vi "EOL Main.vi"() -> ()   [LabVIEW 2018]
uses:
  02.Type Def's/station motion data indicator.ctl
  02.Type Def's/Screen Motion Data.ctl
  02.Type Def's/Pass Fail Control.ctl
  02.Type Def's/station hmi.ctl
  02.Type Def's/lvdt name val pair.ctl
  02.Type Def's/individual station status.ctl
  02.Type Def's/repair station status.ctl
panel:
  in  "NVH Status":bool
  in  "Sunshade Graphs":bool
  out "ms":dbl
  out "All Stations Stopped":bool
  in  "st3":bool
  in  "st0":bool
  in  "O'Scope Data":bool
  in  "Pretty Graphs":bool
  in  "Barcode":bool
  in  "st2":bool
  in  "st1":bool
  in  "All Stations":bool
  in  "Configuration":bool
  in  "Exit Program":bool
  out "Time":string
  out "Date":string
  in  "Main Tab Control":T1(tab)
  in  "Red-Rabbit Mode 3":bool
  in  "Route to Repair st 3":bool
  in  "Abort Test st 3":bool
  in  "Start Test st 3":bool
  in  "Manual Control st 3":bool
  out "all station status st 0":T2={"Error Table Br"=[], "Pass / Fail"=9868950, "Cycle Time Br"=0.0, "Sunroof Barcode"="", "Pallet Number"="", "Part Type"="", "Current Step Br"="", "Application Status"="", "Station Name"="", "Database LVDT's Data Out"=[], "NVH System"=FALSE, "Date"="", "Time"=""} {"Database LVDT's Data Out"."value" format="%.2f"; "Cycle Time Br" format="%#.2g"}
  out "all station status st 3":T2={"Error Table Br"=[], "Pass / Fail"=9868950, "Cycle Time Br"=0.0, "Sunroof Barcode"="", "Pallet Number"="", "Part Type"="", "Current Step Br"="", "Application Status"="", "Station Name"="", "Database LVDT's Data Out"=[], "NVH System"=FALSE, "Date"="", "Time"=""} {"Database LVDT's Data Out"."value" format="%.2f"; "Cycle Time Br" format="%#.2g"}
  in  "Red-Rabbit Mode 2":bool
  in  "Route to Repair st 2":bool
  in  "Abort Test st 2":bool
  in  "Start Test st 2":bool
  in  "Manual Control st 2":bool
  out "all station status st 2":T2={"Error Table Br"=[], "Pass / Fail"=9868950, "Cycle Time Br"=0.0, "Sunroof Barcode"="", "Pallet Number"="", "Part Type"="", "Current Step Br"="", "Application Status"="", "Station Name"="", "Database LVDT's Data Out"=[], "NVH System"=FALSE, "Date"="", "Time"=""} {"Database LVDT's Data Out"."value" format="%.2f"; "Cycle Time Br" format="%#.2g"}
  in  "Red-Rabbit Mode 1":bool
  in  "Route to Repair st 1":bool
  in  "Abort Test st 1":bool
  in  "Start Test st 1":bool
  in  "Manual Control st 1":bool
  in  "Red-Rabbit Mode 0":bool
  out "Repair Station:":T4
  out "Main Title":string=" - All Stations Status"
  in  "Route to Repair st 0":bool
  in  "Abort Test st 0":bool
  in  "Start Test st 0":bool
  in  "Manual Control st 0":bool
  in  "Start Test Re":bool
  in  "Manual Control Repair":bool
  out "all station status st 1":T2={"Error Table Br"=[], "Pass / Fail"=9868950, "Cycle Time Br"=0.0, "Sunroof Barcode"="", "Pallet Number"="", "Part Type"="", "Current Step Br"="", "Application Status"="", "Station Name"="", "Database LVDT's Data Out"=[], "NVH System"=FALSE, "Date"="", "Time"=""} {"Database LVDT's Data Out"."value" format="%.2f"; "Cycle Time Br" format="%#.2g"}
  in  "Tab Control 0":enum32{"Motion Current Data", "Motion Data"}(tab)
  out "Waveform Graph st 0":dbl[](graph)
  out "Motion Data st 0":T5={"Shade Close Limits"={"Noise Test"=enum."Not Tested", "Avg Current"=0.0, "Run Time"=0.0, "Speed"=0.0, "Position"=enum."Not Tested"}, "Shade Close Data 2"={"Noise Test"=enum."Not Tested", "Avg Current"=0.0, "Run Time"=0.0, "Speed"=0.0, "Position"=enum."Not Tested"}, "Shade Open Limits"={"Noise Test"=enum."Not Tested", "Avg Current"=5.0, "Run Time"=5.0, "Speed"=0.0, "Position"=enum."Not Tested"}, "Shade Open Data"={"Noise Test"=enum."Not Tested", "Avg Current"=0.0, "Run Time"=0.0, "Speed"=0.0, "Position"=enum."Not Tested"}, "Vent Close Limits"={"Noise Test"=enum."Not Tested", "Avg Current"=0.0, "Run Time"=0.0, "Speed"=0.0, "Position"=enum."Not Tested"}, "Vent Close Data"={"Noise Test"=enum."Not Tested", "Avg Current"=0.0, "Run Time"=0.0, "Speed"=0.0, "Position"=enum."Not Tested"}, "Vent Open Limits"={"Noise Test"=enum."Not Tested", "Avg Current"=0.0, "Run Time"=0.0, "Speed"=0.0, "Position"=enum."Not Tested"}, "Vent Open Data"={"Noise Test"=enum."Not Tested", "Avg Current"=0.0, "Run Time"=0.0, "Speed"=0.0, "Position"=enum."Not Tested"}, "Slide Close Limits"={"Noise Test"=enum."Not Tested", "Avg Current"=0.0, "Run Time"=0.0, "Speed"=0.0, "Position"=enum."Not Tested"}, "Slide Close Data"={"Noise Test"=enum."Not Tested", "Avg Current"=0.0, "Run Time"=0.0, "Speed"=0.0, "Position"=enum."Not Tested"}, "Slide Open Limits"={"Noise Test"=enum."Not Tested", "Avg Current"=0.0, "Run Time"=0.0, "Speed"=0.0, "Position"=enum."Not Tested"}, "Slide Open Data"={"Noise Test"=enum."Not Tested", "Avg Current"=0.0, "Run Time"=0.0, "Speed"=0.0, "Position"=enum."Not Tested"}} {"Shade Close Limits"."Speed" format="%.2g"; "Shade Close Limits"."Run Time" format="%.2g"; "Shade Close Limits"."Avg Current" format="%.2g"; "Shade Close Data 2"."Speed" format="%.2g"; "Shade Close Data 2"."Run Time" format="%.2g"; "Shade Close Data 2"."Avg Current" format="%.2g"; "Shade Open Limits"."Speed" format="%.2g"; "Shade Open Limits"."Run Time" format="%.2g"; "Shade Open Limits"."Avg Current" format="%.2g"; "Shade Open Data"."Speed" format="%.2g"; "Shade Open Data"."Run Time" format="%.2g"; "Shade Open Data"."Avg Current" format="%.2g"; "Vent Close Limits"."Speed" format="%.2g"; "Vent Close Limits"."Run Time" format="%.2g"; "Vent Close Limits"."Avg Current" format="%.2g"; "Vent Close Data"."Speed" format="%.2g"; "Vent Close Data"."Run Time" format="%.2g"; "Vent Close Data"."Avg Current" format="%.2g"; "Vent Open Limits"."Speed" format="%.2g"; "Vent Open Limits"."Run Time" format="%.2g"; "Vent Open Limits"."Avg Current" format="%.2g"; "Vent Open Data"."Speed" format="%.2g"; "Vent Open Data"."Run Time" format="%.2g"; "Vent Open Data"."Avg Current" format="%.2g"; "Slide Close Limits"."Speed" format="%.2g"; "Slide Close Limits"."Run Time" format="%.2g"; "Slide Close Limits"."Avg Current" format="%.2g"; "Slide Close Data"."Speed" format="%.2g"; "Slide Close Data"."Run Time" format="%.2g"; "Slide Close Data"."Avg Current" format="%.2g"; "Slide Open Limits"."Speed" format="%.2g"; "Slide Open Limits"."Run Time" format="%.2g"; "Slide Open Limits"."Avg Current" format="%.2g"; "Slide Open Data"."Speed" format="%.2g"; "Slide Open Data"."Run Time" format="%.2g"; "Slide Open Data"."Avg Current" format="%.2g"}
  out "Individual Station Status st 0":T8
  in  "Tab Control 1":enum32{"Motion Current Data", "Motion Data"}(tab)
  out "Waveform Graph st 1":dbl[](graph)
  out "Motion Data st 1":T5 {"Shade Close Limits"."Speed" format="%.2g"; "Shade Close Limits"."Run Time" format="%.2g"; "Shade Close Limits"."Avg Current" format="%.2g"; "Shade Close Data 2"."Speed" format="%.2g"; "Shade Close Data 2"."Run Time" format="%.2g"; "Shade Close Data 2"."Avg Current" format="%.2g"; "Shade Open Limits"."Speed" format="%.2g"; "Shade Open Limits"."Run Time" format="%.2g"; "Shade Open Limits"."Avg Current" format="%.2g"; "Shade Open Data"."Speed" format="%.2g"; "Shade Open Data"."Run Time" format="%.2g"; "Shade Open Data"."Avg Current" format="%.2g"; "Vent Close Limits"."Speed" format="%.2g"; "Vent Close Limits"."Run Time" format="%.2g"; "Vent Close Limits"."Avg Current" format="%.2g"; "Vent Close Data"."Speed" format="%.2g"; "Vent Close Data"."Run Time" format="%.2g"; "Vent Close Data"."Avg Current" format="%.2g"; "Vent Open Limits"."Speed" format="%.2g"; "Vent Open Limits"."Run Time" format="%.2g"; "Vent Open Limits"."Avg Current" format="%.2g"; "Vent Open Data"."Speed" format="%.2g"; "Vent Open Data"."Run Time" format="%.2g"; "Vent Open Data"."Avg Current" format="%.2g"; "Slide Close Limits"."Speed" format="%.2g"; "Slide Close Limits"."Run Time" format="%.2g"; "Slide Close Limits"."Avg Current" format="%.2g"; "Slide Close Data"."Speed" format="%.2g"; "Slide Close Data"."Run Time" format="%.2g"; "Slide Close Data"."Avg Current" format="%.2g"; "Slide Open Limits"."Speed" format="%.2g"; "Slide Open Limits"."Run Time" format="%.2g"; "Slide Open Limits"."Avg Current" format="%.2g"; "Slide Open Data"."Speed" format="%.2g"; "Slide Open Data"."Run Time" format="%.2g"; "Slide Open Data"."Avg Current" format="%.2g"}
  out "Individual Station Status st 1":T8
  in  "Tab Control 2":enum32{"Motion Current Data", "Motion Data"}(tab)
  out "Waveform Graph st 2":dbl[](graph)
  out "Motion Data st 2":T5={"Shade Close Limits"={"Noise Test"=enum."Not Tested", "Avg Current"=0.0, "Run Time"=0.0, "Speed"=0.0, "Position"=enum."Not Tested"}, "Shade Close Data 2"={"Noise Test"=enum."Not Tested", "Avg Current"=0.0, "Run Time"=0.0, "Speed"=0.0, "Position"=enum."Not Tested"}, "Shade Open Limits"={"Noise Test"=enum."Not Tested", "Avg Current"=5.0, "Run Time"=5.0, "Speed"=0.0, "Position"=enum."Not Tested"}, "Shade Open Data"={"Noise Test"=enum."Not Tested", "Avg Current"=0.0, "Run Time"=0.0, "Speed"=0.0, "Position"=enum."Not Tested"}, "Vent Close Limits"={"Noise Test"=enum."Not Tested", "Avg Current"=0.0, "Run Time"=0.0, "Speed"=0.0, "Position"=enum."Not Tested"}, "Vent Close Data"={"Noise Test"=enum."Not Tested", "Avg Current"=0.0, "Run Time"=0.0, "Speed"=0.0, "Position"=enum."Not Tested"}, "Vent Open Limits"={"Noise Test"=enum."Not Tested", "Avg Current"=0.0, "Run Time"=0.0, "Speed"=0.0, "Position"=enum."Not Tested"}, "Vent Open Data"={"Noise Test"=enum."Not Tested", "Avg Current"=0.0, "Run Time"=0.0, "Speed"=0.0, "Position"=enum."Not Tested"}, "Slide Close Limits"={"Noise Test"=enum."Not Tested", "Avg Current"=0.0, "Run Time"=0.0, "Speed"=0.0, "Position"=enum."Not Tested"}, "Slide Close Data"={"Noise Test"=enum."Not Tested", "Avg Current"=0.0, "Run Time"=0.0, "Speed"=0.0, "Position"=enum."Not Tested"}, "Slide Open Limits"={"Noise Test"=enum."Not Tested", "Avg Current"=0.0, "Run Time"=0.0, "Speed"=0.0, "Position"=enum."Not Tested"}, "Slide Open Data"={"Noise Test"=enum."Not Tested", "Avg Current"=0.0, "Run Time"=0.0, "Speed"=0.0, "Position"=enum."Not Tested"}} {"Shade Close Limits"."Speed" format="%.2g"; "Shade Close Limits"."Run Time" format="%.2g"; "Shade Close Limits"."Avg Current" format="%.2g"; "Shade Close Data 2"."Speed" format="%.2g"; "Shade Close Data 2"."Run Time" format="%.2g"; "Shade Close Data 2"."Avg Current" format="%.2g"; "Shade Open Limits"."Speed" format="%.2g"; "Shade Open Limits"."Run Time" format="%.2g"; "Shade Open Limits"."Avg Current" format="%.2g"; "Shade Open Data"."Speed" format="%.2g"; "Shade Open Data"."Run Time" format="%.2g"; "Shade Open Data"."Avg Current" format="%.2g"; "Vent Close Limits"."Speed" format="%.2g"; "Vent Close Limits"."Run Time" format="%.2g"; "Vent Close Limits"."Avg Current" format="%.2g"; "Vent Close Data"."Speed" format="%.2g"; "Vent Close Data"."Run Time" format="%.2g"; "Vent Close Data"."Avg Current" format="%.2g"; "Vent Open Limits"."Speed" format="%.2g"; "Vent Open Limits"."Run Time" format="%.2g"; "Vent Open Limits"."Avg Current" format="%.2g"; "Vent Open Data"."Speed" format="%.2g"; "Vent Open Data"."Run Time" format="%.2g"; "Vent Open Data"."Avg Current" format="%.2g"; "Slide Close Limits"."Speed" format="%.2g"; "Slide Close Limits"."Run Time" format="%.2g"; "Slide Close Limits"."Avg Current" format="%.2g"; "Slide Close Data"."Speed" format="%.2g"; "Slide Close Data"."Run Time" format="%.2g"; "Slide Close Data"."Avg Current" format="%.2g"; "Slide Open Limits"."Speed" format="%.2g"; "Slide Open Limits"."Run Time" format="%.2g"; "Slide Open Limits"."Avg Current" format="%.2g"; "Slide Open Data"."Speed" format="%.2g"; "Slide Open Data"."Run Time" format="%.2g"; "Slide Open Data"."Avg Current" format="%.2g"}
  out "Individual Station Status st 2":T8
  out "Sunshade Servo Data Open":dbl[](graph)
  out "AP Data Graph":i16[][](graph)
  in  "AP Data":path
  in  "Update AP Data":bool
  out "Sunshade Servo Data Close":dbl[](graph)
  out "Individual Station Status st 3":T8
  in  "Tab Control 3":enum32{"Motion Current Data", "Motion Data"}(tab)
  out "Waveform Graph st 3":dbl[](graph)
  out "Motion Data st 3":T5 {"Shade Close Limits"."Speed" format="%.2g"; "Shade Close Limits"."Run Time" format="%.2g"; "Shade Close Limits"."Avg Current" format="%.2g"; "Shade Close Data 2"."Speed" format="%.2g"; "Shade Close Data 2"."Run Time" format="%.2g"; "Shade Close Data 2"."Avg Current" format="%.2g"; "Shade Open Limits"."Speed" format="%.2g"; "Shade Open Limits"."Run Time" format="%.2g"; "Shade Open Limits"."Avg Current" format="%.2g"; "Shade Open Data"."Speed" format="%.2g"; "Shade Open Data"."Run Time" format="%.2g"; "Shade Open Data"."Avg Current" format="%.2g"; "Vent Close Limits"."Speed" format="%.2g"; "Vent Close Limits"."Run Time" format="%.2g"; "Vent Close Limits"."Avg Current" format="%.2g"; "Vent Close Data"."Speed" format="%.2g"; "Vent Close Data"."Run Time" format="%.2g"; "Vent Close Data"."Avg Current" format="%.2g"; "Vent Open Limits"."Speed" format="%.2g"; "Vent Open Limits"."Run Time" format="%.2g"; "Vent Open Limits"."Avg Current" format="%.2g"; "Vent Open Data"."Speed" format="%.2g"; "Vent Open Data"."Run Time" format="%.2g"; "Vent Open Data"."Avg Current" format="%.2g"; "Slide Close Limits"."Speed" format="%.2g"; "Slide Close Limits"."Run Time" format="%.2g"; "Slide Close Limits"."Avg Current" format="%.2g"; "Slide Close Data"."Speed" format="%.2g"; "Slide Close Data"."Run Time" format="%.2g"; "Slide Close Data"."Avg Current" format="%.2g"; "Slide Open Limits"."Speed" format="%.2g"; "Slide Open Limits"."Run Time" format="%.2g"; "Slide Open Limits"."Avg Current" format="%.2g"; "Slide Open Data"."Speed" format="%.2g"; "Slide Open Data"."Run Time" format="%.2g"; "Slide Open Data"."Avg Current" format="%.2g"}
  in  "Tab Control 4":enum32{"Motion Current Data", "Motion Data"}(tab)
  # "EOL v4.3.4.0"
  # "Sunroof Barcode"
  # "Pallet Number"
  # "Part Type"
  # "Application Status"
  # "Current Step"
  # "Cycle Time"
  # "Pass / Fail"
  # "Sunroof Barcode"
  # "Pallet Number"
  # "Part Type"
  # "Application Status"
  # "Current Step"
  # "Cycle Time"
  # "Pass / Fail"
  # "Sunroof Barcode"
  # "Pallet Number"
  # "Part Type"
  # "Application Status"
  # "Current Step"
  # "Cycle Time"
  # "Pass / Fail"
  # "Part Type"
  # "Application Status"
  # "Pallet Number"
  # "Sunroof Barocde"
  # "Sunroof Barcode"
  # "Pallet Number"
  # "Part Type"
  # "Application Status"
  # "Current Step"
  # "Cycle Time"
  # "Pass / Fail"
  # "Shade Close"
  # "Actual Data"
  # "Limits"
  # "Avg Current"
  # "Run Time"
  # "Speed"
  # "Noise Test"
  # "Position"
  # "Shade Open"
  # "Actual Data"
  # "Limits"
  # "Avg Current"
  # "Run Time"
  # "Speed"
  # "Noise Test"
  # "Position"
  # "Vent Close"
  # "Actual Data"
  # "Limits"
  # "Avg Current"
  # "Run Time"
  # "Speed"
  # "Noise Test"
  # "Position"
  # "Vent Open"
  # "Actual Data"
  # "Limits"
  # "Avg Current"
  # "Run Time"
  # "Speed"
  # "Noise Test"
  # "Position"
  # "Slide Close"
  # "Actual Data"
  # "Limits"
  # "Avg Current"
  # "Run Time"
  # "Speed"
  # "Noise Test"
  # "Position"
  # "Slide Open"
  # "Actual Data"
  # "Limits"
  # "Avg Current"
  # "Run Time"
  # "Speed"
  # "Noise Test"
  # "Position"
  # "Shade Close"
  # "Actual Data"
  # "Limits"
  # "Avg Current"
  # "Run Time"
  # "Speed"
  # "Noise Test"
  # "Position"
  # "Shade Open"
  # "Actual Data"
  # "Limits"
  # "Avg Current"
  # "Run Time"
  # "Speed"
  # "Noise Test"
  # "Position"
  # "Vent Close"
  # "Actual Data"
  # "Limits"
  # "Avg Current"
  # "Run Time"
  # "Speed"
  # "Noise Test"
  # "Position"
  # "Vent Open"
  # "Actual Data"
  # "Limits"
  # "Avg Current"
  # "Run Time"
  # "Speed"
  # "Noise Test"
  # "Position"
  # "Slide Close"
  # "Actual Data"
  # "Limits"
  # "Avg Current"
  # "Run Time"
  # "Speed"
  # "Noise Test"
  # "Position"
  # "Slide Open"
  # "Actual Data"
  # "Limits"
  # "Avg Current"
  # "Run Time"
  # "Speed"
  # "Noise Test"
  # "Position"
  # "Shade Close"
  # "Actual Data"
  # "Limits"
  # "Avg Current"
  # "Run Time"
  # "Speed"
  # "Noise Test"
  # "Position"
  # "Shade Open"
  # "Actual Data"
  # "Limits"
  # "Avg Current"
  # "Run Time"
  # "Speed"
  # "Noise Test"
  # "Position"
  # "Vent Close"
  # "Actual Data"
  # "Limits"
  # "Avg Current"
  # "Run Time"
  # "Speed"
  # "Noise Test"
  # "Position"
  # "Vent Open"
  # "Actual Data"
  # "Limits"
  # "Avg Current"
  # "Run Time"
  # "Speed"
  # "Noise Test"
  # "Position"
  # "Slide Close"
  # "Actual Data"
  # "Limits"
  # "Avg Current"
  # "Run Time"
  # "Speed"
  # "Noise Test"
  # "Position"
  # "Slide Open"
  # "Actual Data"
  # "Limits"
  # "Avg Current"
  # "Run Time"
  # "Speed"
  # "Noise Test"
  # "Position"
  # "Station 60"
  # "Shade Close"
  # "Actual Data"
  # "Limits"
  # "Avg Current"
  # "Run Time"
  # "Speed"
  # "Noise Test"
  # "Position"
  # "Shade Open"
  # "Actual Data"
  # "Limits"
  # "Avg Current"
  # "Run Time"
  # "Speed"
  # "Noise Test"
  # "Position"
  # "Vent Close"
  # "Actual Data"
  # "Limits"
  # "Avg Current"
  # "Run Time"
  # "Speed"
  # "Noise Test"
  # "Position"
  # "Vent Open"
  # "Actual Data"
  # "Limits"
  # "Avg Current"
  # "Run Time"
  # "Speed"
  # "Noise Test"
  # "Position"
  # "Slide Close"
  # "Actual Data"
  # "Limits"
  # "Avg Current"
  # "Run Time"
  # "Speed"
  # "Noise Test"
  # "Position"
  # "Slide Open"
  # "Actual Data"
  # "Limits"
  # "Avg Current"
  # "Run Time"
  # "Speed"
  # "Noise Test"
  # "Position"
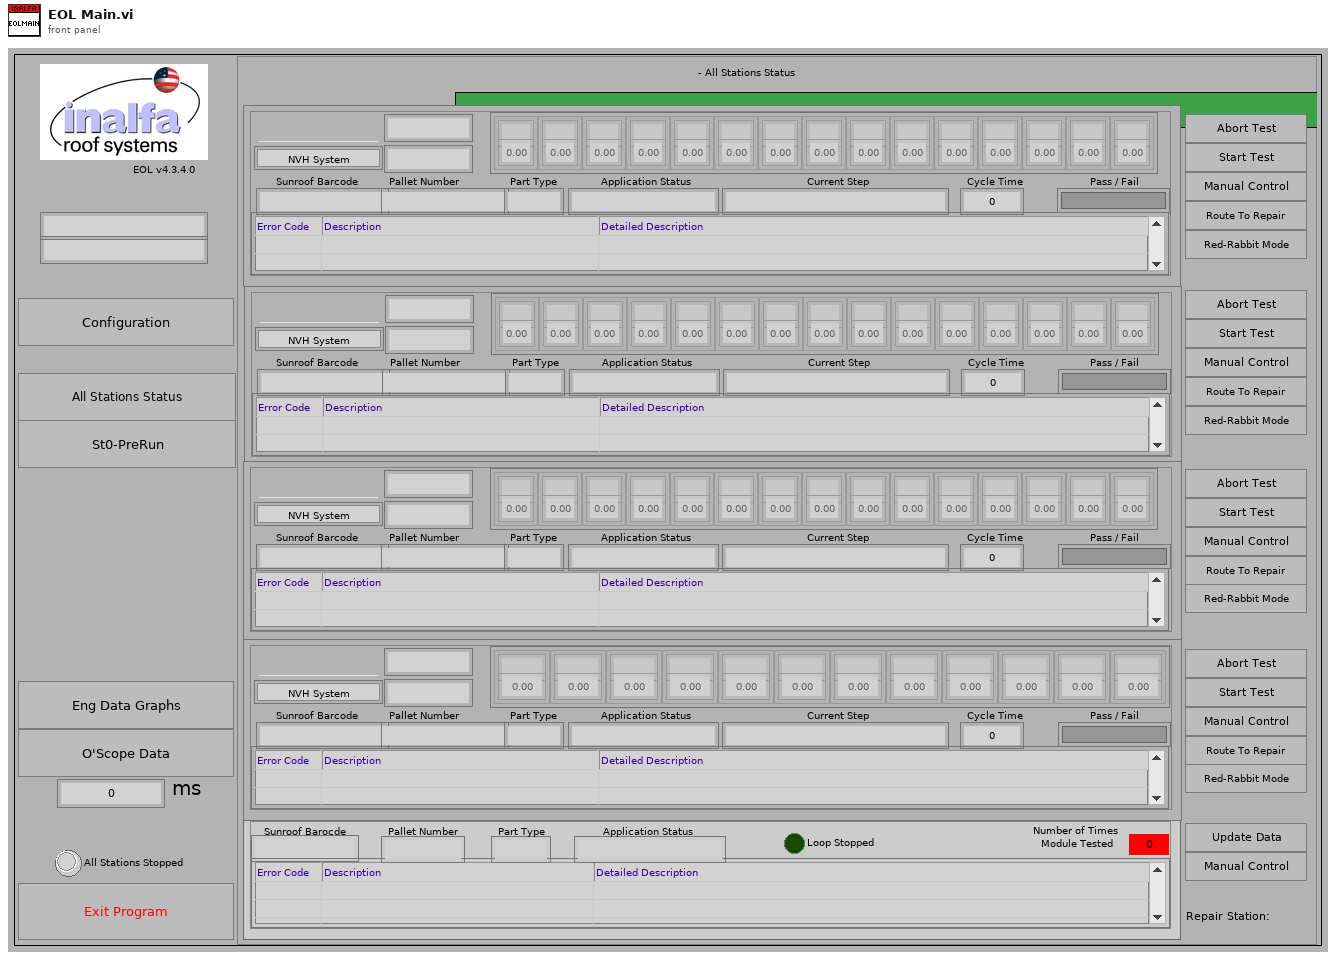
[diagram p1: front panel]
types:
  T1 = enum32{"All Stations Status", "Station 0", "Station 1", "Station 2", "Barcode Station", "Eng Data Graphs", "Station 3", "Station 4"}
  T2 = typedef "station hmi.ctl" = cluster{"Error Table Br":string[][], "Pass / Fail":u32, "Cycle Time Br":dbl, "Sunroof Barcode":string, "Pallet Number":string, "Part Type":string, "Current Step Br":string, "Application Status":string, "Station Name":string, "Database LVDT's Data Out":T3[], "NVH System":bool, "Date":string, "Time":string}
  T3 = typedef "lvdt name val pair.ctl" = cluster{"lvdt name":string, "value":dbl}
  T4 = typedef "repair station status.ctl" = cluster{"Loop Stopped":bool, "Error Table":string[][], "Sunroof Barcode":string, "Pallet Number":string, "Application Status":string, "Part Type":string, "Number of Times\n Module Tested":u8}
  T5 = typedef "station motion data indicator.ctl" = cluster{"Shade Close Limits":T6, "Shade Close Data 2":T6, "Shade Open Limits":T6, "Shade Open Data":T6, "Vent Close Limits":T6, "Vent Close Data":T6, "Vent Open Limits":T6, "Vent Open Data":T6, "Slide Close Limits":T6, "Slide Close Data":T6, "Slide Open Limits":T6, "Slide Open Data":T6}
  T6 = typedef "Screen Motion Data.ctl" = cluster{"Noise Test":T7, "Avg Current":dbl, "Run Time":dbl, "Speed":dbl, "Position":T7}
  T7 = typedef "Pass Fail Control.ctl" = enum16{"Not Tested", "Pass", "Fail"}
  T8 = typedef "individual station status.ctl" = cluster{"Line Number":u8, "Serial Port":bool, "Loop Stopped?":bool, "Nidec Serial #":string, "Platform Constant":string, "ATS Constant":string, "Position Constant":string, "Schematic Ver":string, "Bootloader Ver":string, "Hardware Ver":string, "Vehicle Type":string, "Inalfa Motor P/N":string, "System Mode":string, "DTC's?":bool, "Calibrated?":bool, "Slide Count":u16, "Vent Count":u16, "Glass Voltage":dbl, "Anti Pinch Test?":bool, "Station":string}
  T9 = typedef "main state cluster.ctl" = cluster{"Application Status":string, "Switch Output Array":T10[], "Switch Value Configuration":T12[], "NVH Configuration":T14, "rs232 port map":T15, "ethernet address map":T16, "paths":T17, "Station Index":i32, "Store Data":T18, "D in map":T24, "DO Task":refnum<k21>, "ctl refs":T26, "misc station config":T27, "ethernet tcp refs":cluster{"LVDT Unit":refnum<k5>}, "Sunshade Barcode Scan":cluster{"Sunshade Number 2":string, "Sunshade Number 1":string, "Keyence tuning bank idx":i32}, "AP Test Data":cluster{"Raw Sunshade AP Data":string, "Raw Glass AP Data":string, "PMAC Read Counter":dbl, "Database AP Data":dbl[]}, "Motion Status":cluster{"hmi operator abort start time":u32, "Current Data Index":i32, "Analog Data":sgl[][], "Motor Position Hex":u16, "Messages Index":u16, "Last Bytes":u8[], "Current Hall Position":i16, "Motion Stop Timer":u32, "Position Test":T7, "Noise Test":T7, "motion stop check initialized":bool, "remote sense enabled":bool, "Motion":T11}, "LVDT Status":cluster{"LVDT's stored config":T29[], "lvdt precision":T30}, "Sequence State":T31, "misc status":cluster{"delay start time (ticks)":u32, "In Vehicle Mode?":bool, "Diag Mode?":bool, "Serial Port Configured?":bool, "PS Voltage":dbl, "Diag Serial Port":refnum<visa-resource-name>, "Part Setup":T33, "Part History Number":string, "Plant Number":u8, "AP Data Type":T21, "Real Rollo?":bool}, "NVH Operator?":bool, "NVH Pass?":bool, "Operator Pass?":bool, "Operator Action?":bool, "Noise Source":u32, "USBHandle":i32, "PeakInfo":string, "PeakNumber":i32, "NVH Motion Steps":string[], "Second Check?":bool, "Decibel data":dbl[], "Direct Control Info":cluster{"EnableStopOnHome":bool, "EnableStopOnPos":bool, "TeachEvent":bool, "open offset":i32, "close offset":i32, "Derect control":bool, "set position":i32[], "teach pass ":bool, "Drift offsets":i32[], "Hall Positions":i32[]}, "manual control(direct)":bool, "LIN INFO":T38, "Config Info":T41}
  T10 = typedef "All Switch Configuration Cluster.ctl" = cluster{"All Motions":T11, "A":bool[], "B":bool[], "C":bool[], "D":bool[], "A activation time (ms)":u32, "B activation time (ms)":u32, "C activation time (ms)":u32}
  T11 = typedef "All Motions.ctl" = enum16{"Glass Teach", "Glass Slide Open", "Glass Slide Close", "Glass Vent Open", "Glass Vent Close", "Sunshade Teach", "Sunshade Open", "Sunshade Close", "Idle", "Sunshade Open 2", "Sunshade Close 2", "Glass Slide Open Sunshade Open", "Glass Slide Open Sunshade Close", "Glass Slide Close Sunshade Open", "Glass Slide Close Sunshade Close", "Glass Vent Open Sunshade Open", "Glass Vent Open Sunshade Close", "Glass Vent Close Sunshade Open", "Glass Vent Close Sunshade Close", "Express Glass Slide Open", "Express Glass Slide Close", "Express Glass Vent Open", "Express Glass Vent Close", "Express Sunshade Open", "Express Sunshade Close", "Express Sunshade Open 2", "Express Sunshade Close 2", "Express Glass Slide Open Sunshade Open", "Express Glass Slide Open Sunshade Close", "Express Glass Slide Close Sunshade Open", "Express Glass Slide Close Sunshade Close", "Express Glass Vent Open Sunshade Open", "Express Glass Vent Open Sunshade Close", "Express Glass Vent Close Sunshade Open", "Express Glass Vent Close Sunshade Close", "Goto Position Glass", "Goto Position Sunshade", "Sunshade Teach 2"}
  T12 = typedef "EOL Switch Value Configuration Cluster.ctl" = cluster{"All Motions":T11, "Array":T13[]}
  T13 = typedef "EOL Switch Max Min Check Cluster.ctl" = cluster{"Min":dbl, "Max":dbl, "Check?":bool}
  T14 = typedef "station nvh config.ctl" = cluster{"NVH Station?":bool, "nvh app instance path":string, "NVH_ErrorMessages sv url":string, "NVH_Inputs sv url":string, "NVH_MotionNumber sv url":string, "NVH_Outputs sv url":string, "NVH_PartNumber sv url":string, "NVH_PartNumber_Echo sv url":string, "NVH_SerialNumber sv url":string, "NVH_AmbientTempF sv url":string}
  T15 = typedef "station rs232 port map.ctl" = cluster{"PMAC":refnum<visa-resource-name>, "PS Port":refnum<visa-resource-name>, "LVDT Unit":refnum<visa-resource-name>, "RS232":refnum<visa-resource-name>}
  T16 = typedef "station ethernet address map.ctl" = cluster{"LVDT 1 Unit":string, "LVDT Unit 1 port":u16}
  T17 = typedef "station paths.ctl" = cluster{"Base Path":path, "system error log path":path, "Error Table Path":path, "Store errors log path":path, "data bytes log path":path, "network path":path}
  T18 = typedef "EOL Save Module Test Data Control.ctl" = cluster{"Motion Data Array":T19[], "Error Table":string[][], "Sun Shade Close Force Limits":T22, "Sun Shade Open Force Limits":T22, "Sunshade Open Data":sgl[], "Sunshade Close Data":sgl[], "Module Info":T23, "Sunsahde Close Raw Data":sgl[], "Sunshade Open Raw Data":sgl[], "Software Version":string[], "Constant Version":string[], "Hardware Version":string[], "Inalfa Part Number ECU":string[], "LVDT Data":sgl[], "Communication Line 1":sgl[], "Communication Line 2":sgl[], "Anti Pinch Force":sgl[], "Cycle Time":string, "Anti Pinch Vent Force":sgl[], "iGPS LVDT Data":sgl[], "data bytes log":string}
  T19 = typedef "EOL Motion Database Table.ctl" = cluster{"Motion":T11, "Actual Avg Current":dbl, "Actual Runtime":dbl, "Actual Speed":dbl, "Current Data":sgl[], "Motion Data Limits":T20, "Switch 1 to 6":dbl[], "Actual PS Voltage":dbl, "AP Data":i16[][], "Actual max Current":dbl, "Actual Noise (dB)":dbl}
  T20 = typedef "17x Audit Motion Data Seq Control.ctl" = cluster{"Power Supply Voltage":dbl, "Min Avg Current":dbl, "Max Avg Current":dbl, "Min Run Time":dbl, "Max Run Time":dbl, "Min Speed":dbl, "Max Speed":dbl, "AP Data % of Threshold":dbl, "Travel Distance":dbl, "AP Data Type":T21, "Check Current":bool, "Check Run Time":bool, "Check Speed":bool, "Express Motion?":bool, "Check Sound Test":bool, "Check Position?":bool, "Collect AP Data":bool, "Inital Position":u16, "End Position":u16, "Goto Posiition":u16, "Max max Current":dbl, "Min max Current":dbl, "Check max Current":bool, "Check Sound":bool, "Min Sound (dB)":dbl, "Max Sound (dB)":dbl, "SW Mode":enum16{"Hard Switch", "Uncond Frame"}, "LIN Msg":cluster{"ID":u8, "Msg":u8[][], "LDF":refnum<k21>}}
  T21 = typedef "17x AP Data Type.ctl" = enum16{"91/61", "92/62", "93/63", "67", "68", "6F", "71", "91 Msg", "92 Msg", "93 Msg", "94 Msg", "HiRain 91", "HiRain 92 Speed", "HiRain 92 HS", "HiRain 92", "HiRain 93", "SnT"}
  T22 = typedef "17x Sunshade Limts Seq.ctl" = cluster{"Overall Min":dbl, "Overall Max":dbl, "Avg Min":dbl, "Avg Max":dbl, "Truncation Start":dbl, "Truncation End":dbl, "Variance":dbl, "Check Noise":bool}
  T23 = typedef "EOL Module Info Control.ctl" = cluster{"Serial Number":string, "Pallet Number":string, "Sunshade Color":string, "Inalfa Part Number":string, "Customer Number":string}
  T24 = typedef "station DI map.ctl" = cluster{"Abort Test":T25, "Start Test":T25}
  T25 = typedef "EOL Global Digital Input Control.ctl" = enum16{"Dev2/port0/line0", "Dev2/port0/line1", "Dev2/port0/line2", "Dev2/port0/line3", "Dev2/port0/line4", "Dev2/port0/line5", "Dev2/port0/line6", "Dev2/port0/line7", "Dev2/port1/line0", "Dev2/port1/line1", "Dev2/port1/line2", "Dev2/port1/line3", "Dev2/port1/line4", "Dev2/port1/line5", "Dev2/port1/line6", "Dev2/port1/line7", "Dev2/port2/line0", "Dev2/port2/line1", "Dev2/port2/line2", "Dev2/port2/line3", "Dev2/port2/line4", "Dev2/port2/line5", "Dev2/port2/line6", "Dev2/port2/line7", "Prerun Start Test", "Prerun Abort Test", "Audit Start Test", "Audit Abort Test", "Dev2/port3/line4", "Dev2/port3/line5", "Breakin Start Test", "Breakin Abort Test", "Not Implemented"}
  T26 = typedef "control refs.ctl" = cluster{"Start Test":refnum<vi>, "Abort Test":refnum<vi>, "Manual Control":refnum<vi>, "Route to Repair":refnum<vi>, "Waveform Graph":refnum<vi>, "Motion Data":refnum<vi>, "all station status":refnum<vi>, "Individual Station Status":refnum<vi>, "exit program":refnum<vi>, "Sunshade Servo Data Open":refnum<vi>, "Sunshade Servo Data Close":refnum<vi>, "Red-Rabbit Mode":refnum<vi>, "Direct Manual Ctrl":refnum<vi>}
  T27 = typedef "misc station config.ctl" = cluster{"Station Name":string, "is AT station?":bool, "is audit station?":bool, "power supply type":T28, "use alt China TP2 LVDT Logic Seq":bool, "hmi operator abort timeout":u32, "dump all analog values even if pass":bool, "debug log pre-filter ap stream bytes":bool, "use separate lvdt x and z extend tags":bool, "is print":bool}
  T28 = typedef "power supply types.ctl" = enum16{"GENser", "ZUPser", "GENeth", "Manual", "ITECH"}
  T29 = typedef "EOL LVDT's Check Controller.ctl" = cluster{"Upper Limit":dbl, "Lower Limit":dbl, "LVDT Name":string, "Check":bool}
  T30 = typedef "lvdt precision.ctl" = cluster{"truncate instead of rounding":bool, "decimal places":u8}
  T31 = typedef "sequence state.ctl" = cluster{"Step Description":string, "Cycle Start Time":u32, "Step Data String":string, "Pass?":bool, "Seqence":T32[], "Active Step":u8, "Testing?":bool, "Red-Rabbit Mode":bool, "route-to-repair mode":bool, "NVH Status":cluster{"Restart IRQ Counter":u8, "NVH Test Needed?":bool, "NVH Test Running?":bool}, "Present (s)":dbl, "Hold Mode?":bool, "Hold?":bool, "Rx Invalid?":bool}
  T32 = typedef "Sequence Info.ctl" = cluster{"Name":string, "Description":string, "data string":string}
  T33 = typedef "EOL Part Setup.ctl" = cluster{"Communication Type":T34, "Send Messages to":T35, "RAP Signal":T36, "Motor Type":T37, "NVH Part Number":u16, "Turn Off Timer":u16, "Part Type":string}
  T34 = typedef "All Communication Types.ctl" = enum16{"None", "CAN", "RS 232", "RS 232 LIN", "GM LIN", "SnT LIN", "K Line", "Robel CAN", "P42M-Continental", "Inalfa SCU LIN", "Spare 3"}
  T35 = typedef "Communication with Motors.ctl" = enum16{"Glass", "Rollo", "Both"}
  T36 = typedef "RAP Signal Control.ctl" = enum16{"High", "Low", "None"}
  T37 = typedef "EOL Motor Type.ctl" = enum16{"Smart Motor", "Sensor Motor"}
  T38 = typedef "station LIN config.ctl" = cluster{"Toolkit Type":enum16{"Inalfa LIN", "ADCS LIN", "TS LIN"}, "NAD":u8, "Inalfa LIN":T39, "ADCS LIN":T40, "TS LIN":cluster{"ref info":refnum<k24>, "LIN Channel":i32, "ByteCmd Path":path}}
  T39 = typedef "LIN Device.ctl" = cluster{"Master Frame(3C)":refnum<k21>, "Slave Frame(3D)":refnum<k21>, "Request Schedule":refnum<k21>, "Response Schedule":refnum<k21>, "Frame Write SCU":refnum<k21>, "Frame Read SCU":refnum<k21>, "LIN Name":refnum<k21>}
  T40 = typedef "ADCS_LIN info.ctl" = cluster{"Port":string, "HW select":u16, "XNET Cluster":string, "ByteCmd Path":path}
  T41 = typedef "Config Info.ctl" = variant
  T42 = enum32{"All Stations Status", "Station 0", "Station 1", "Station 2", "Barcode Station", "Eng Data Graphs", "Station 3"}
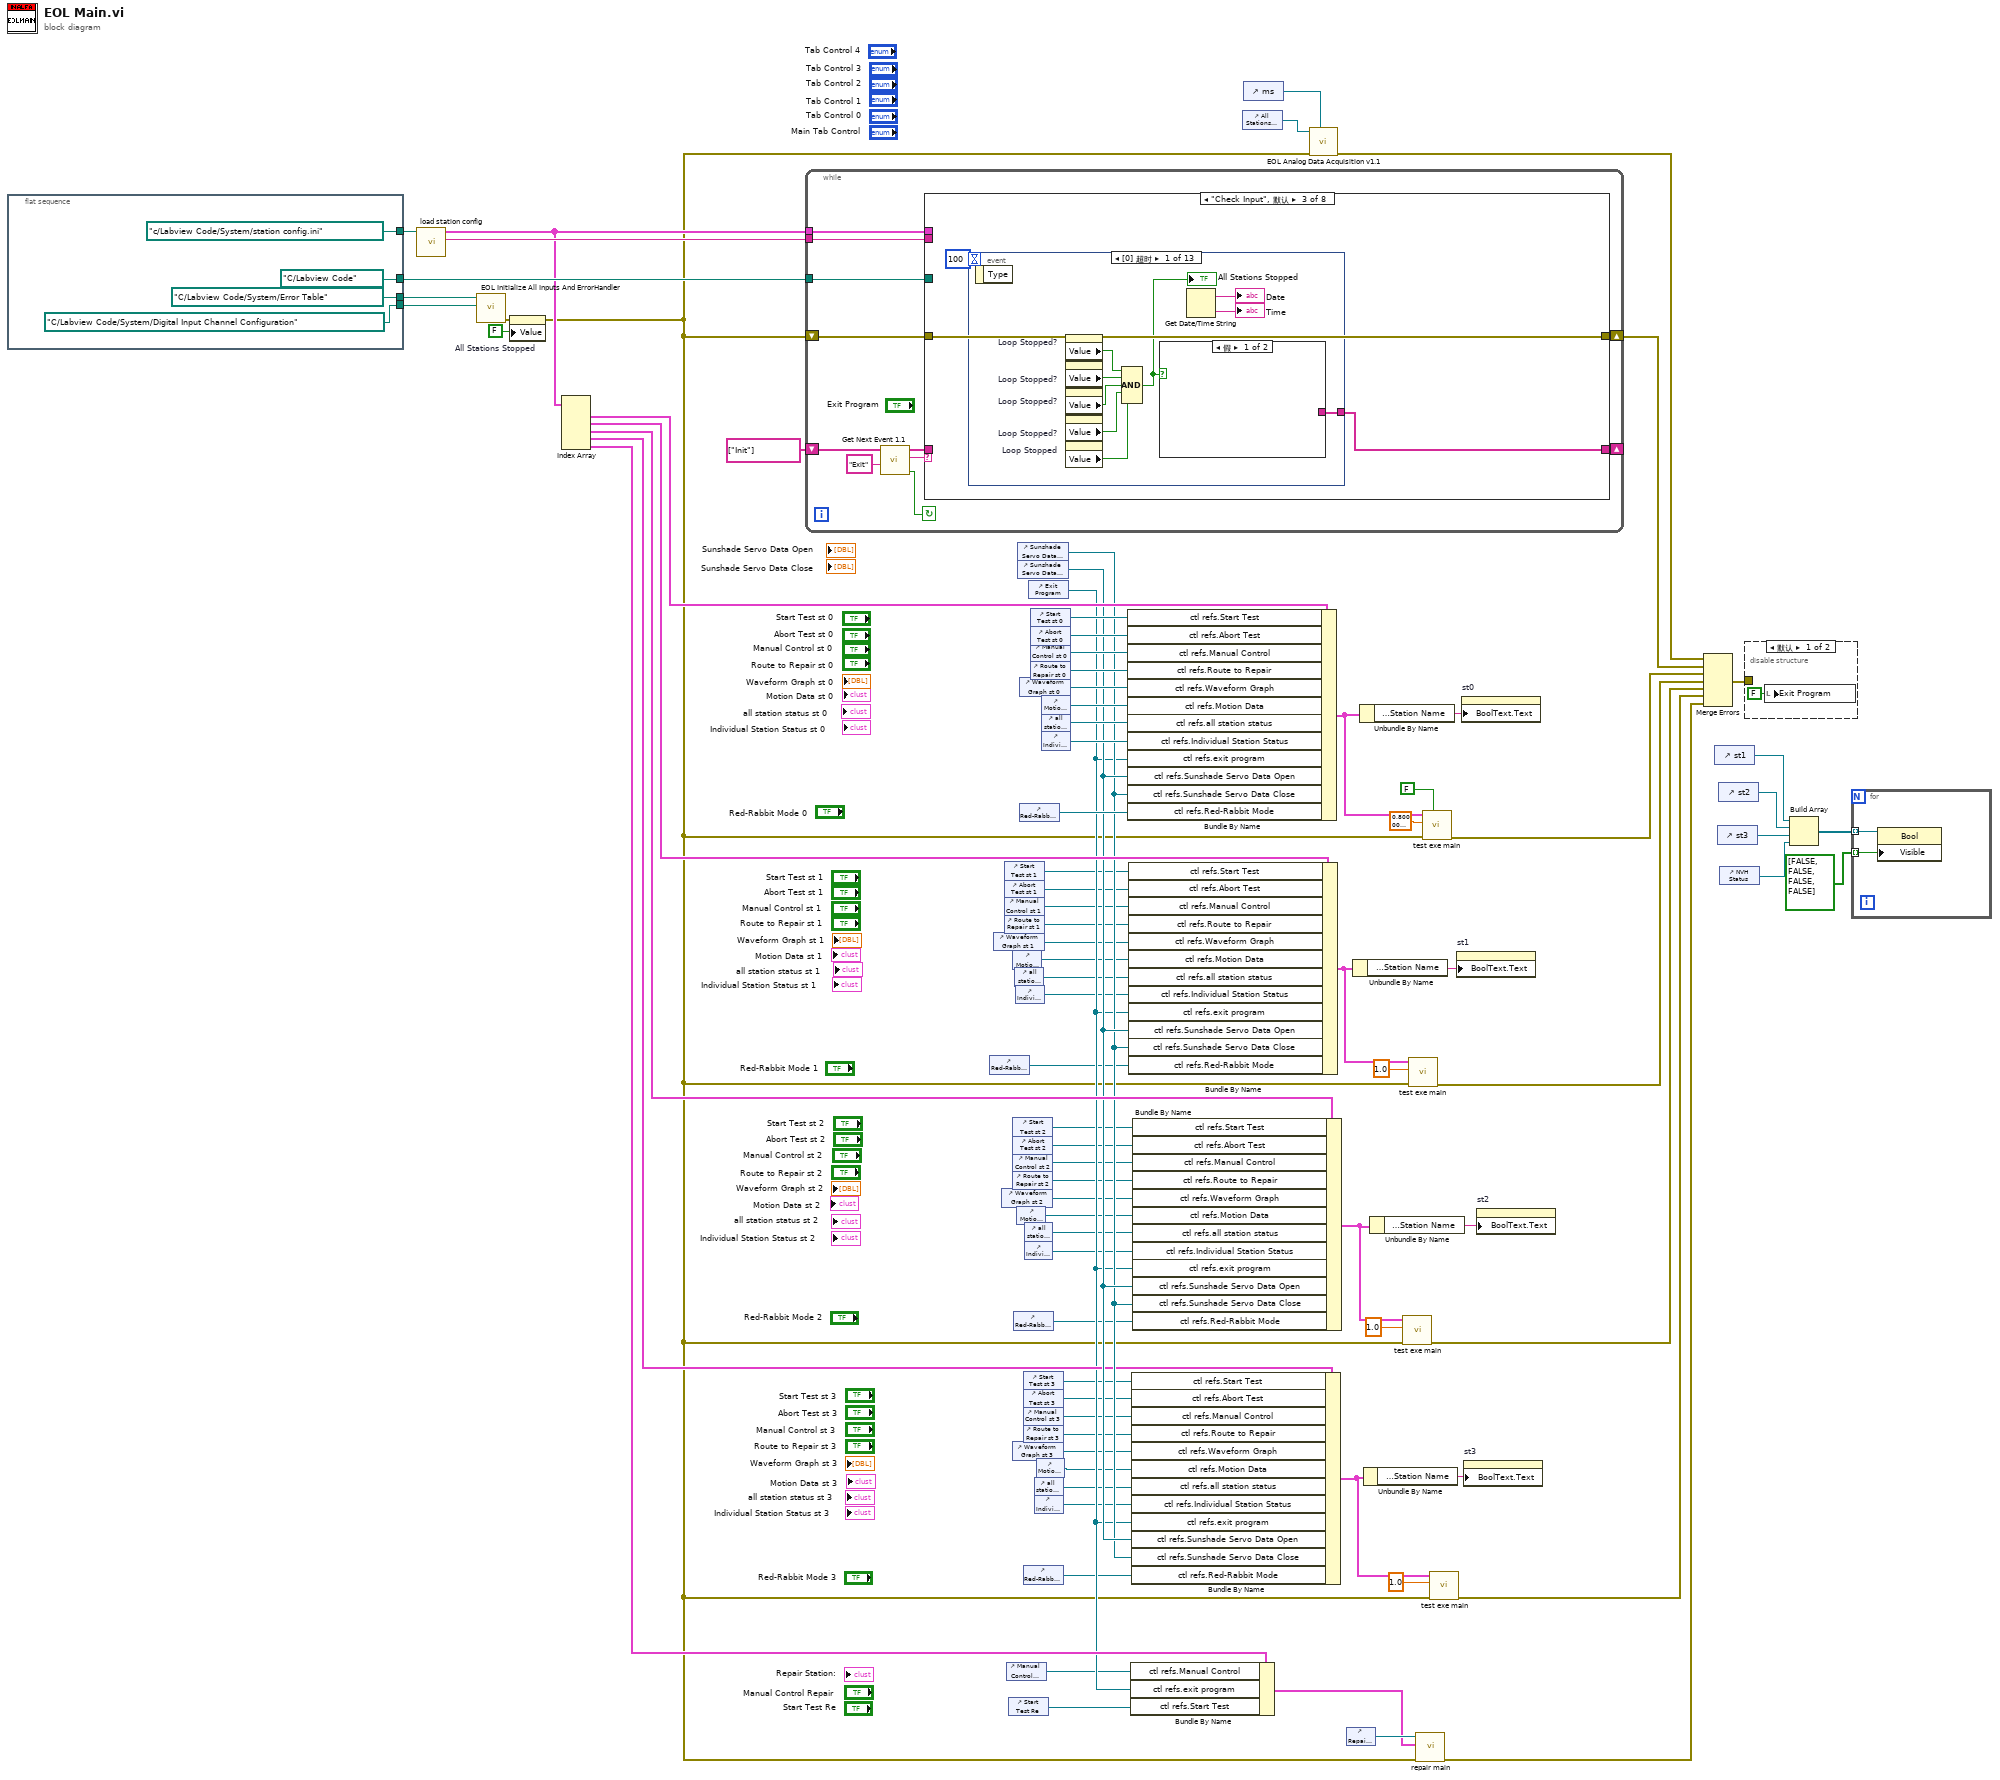
[diagram p0: block diagram]
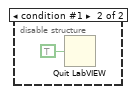
[diagram p2: hidden frame]
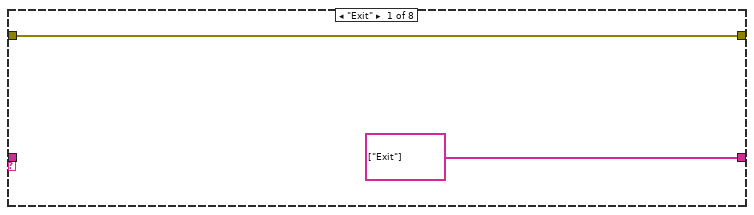
[diagram p3: hidden frame]
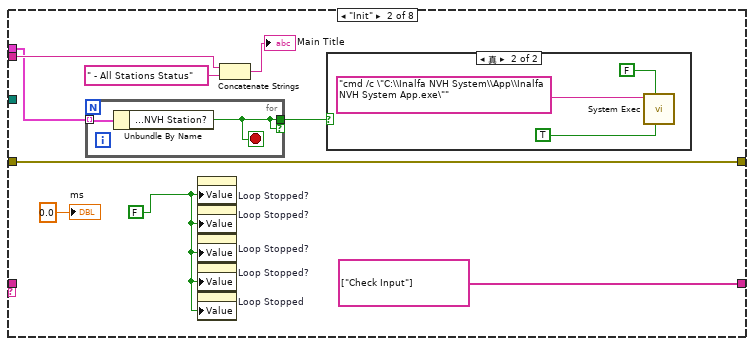
[diagram p4: hidden frame]
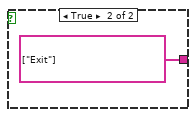
[diagram p6: hidden frame]
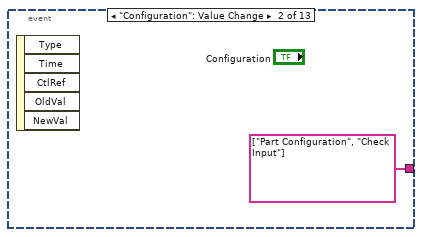
[diagram p7: hidden frame]
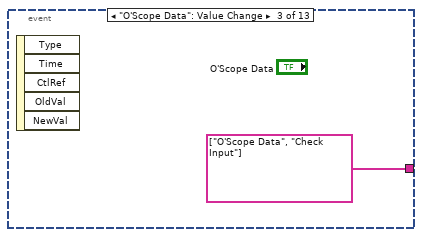
[diagram p8: hidden frame]
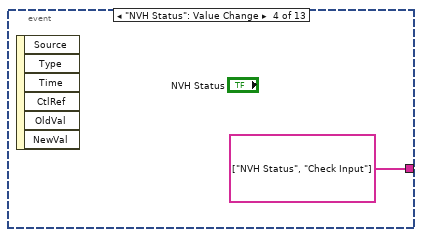
[diagram p9: hidden frame]
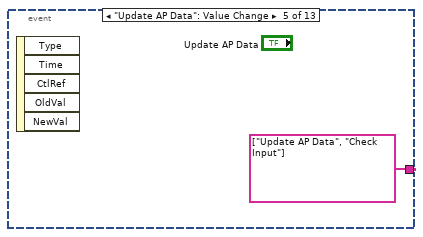
[diagram p10: hidden frame]
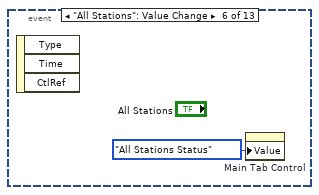
[diagram p11: hidden frame]
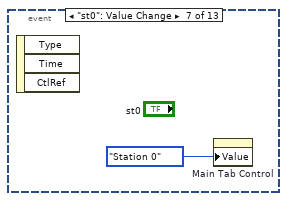
[diagram p12: hidden frame]
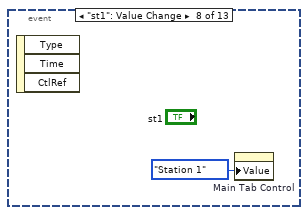
[diagram p13: hidden frame]
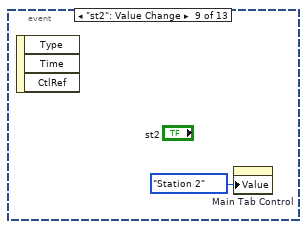
[diagram p14: hidden frame]
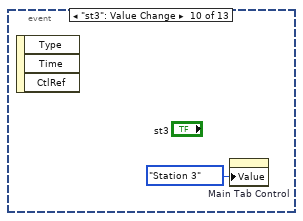
[diagram p15: hidden frame]
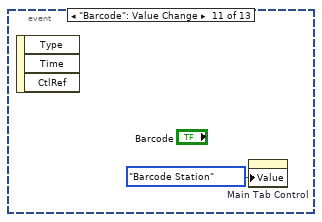
[diagram p16: hidden frame]
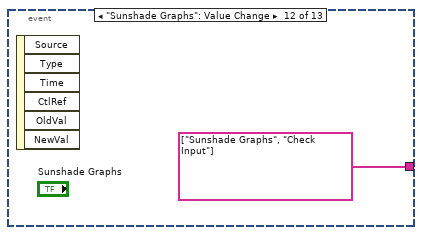
[diagram p17: hidden frame]
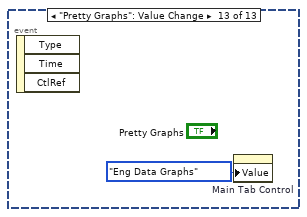
[diagram p18: hidden frame]
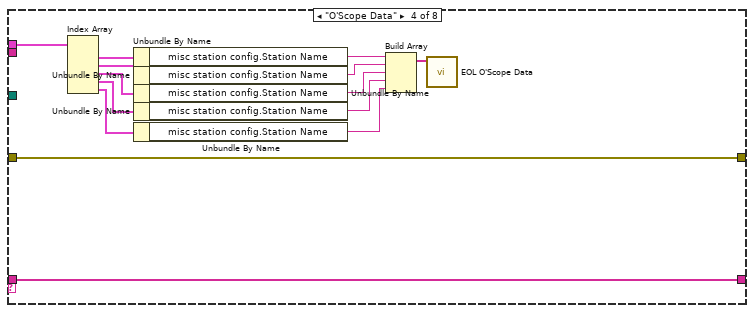
[diagram p19: hidden frame]
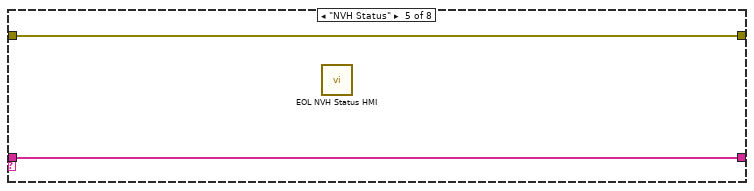
[diagram p20: hidden frame]
diagram:
  n1 = flat-sequence {
    tunnel: [path "C:/Labview Code/System/Error Table" ("Error Table Path")] -> w78
    tunnel: [path "C:/Labview Code/System/Digital Input Channel Configuration" ("DI Map Path")] -> w77
    tunnel: [path "c:/Labview Code/System/station config.ini" ("station config file path")] -> w76
    tunnel: [path "C:/Labview Code" ("Program Root Path")] -> w62
    frame #0 {
    }
  }
  n2 = call "load station config.vi"("station config file path"=w76) -> ("Line Name"=w72:string, "all satation cluster"=w57:T9[])  [unwired: 8 in, 1 out]
  n3 = call "EOL Initialize All Inputs And ErrorHandler.vi"("DI Map Path"=w77, "Error Table Path"=w78) -> ("Sys Error Out"=w71:errorcluster)  [unwired: 9 in]
  n4 = property on="All Stations Stopped" class="Bool (严格)"(error in=w71, "Value"=FALSE ("All Stations Stopped")) -> (error out=w51:errorcluster)  [unwired: 1 in, 1 out]
  n5 = Index Array(array=w57) -> (element #1=w64:T9, element #2=w63:T9, element #3=w58:T9, element #4=w54:T9, element #5=w53:T9)  [unwired: 5 in]
  n6 = while {
    shift-right: [w98] -> _
    shift-left: string[] ["Init"] ("event queue out") -> [w97]
    tunnel: w57 -> [w96]
    shift-right: [w95] -> w73
    shift-left: w51 -> [w92]
    tunnel: w72 -> [w94]
    tunnel: w62 -> [w93]
    stop <- w102 continue-if-true
    n7 = call "Get Next Event 1.1.vi"("Exit Event"="Exit", "event queue in"=w97) -> ("Condition (Exit:F)"=w102:bool, "next event"=w100:string, "event queue out"=w99:string[])  [unwired: 6 in, 1 out]
    n8 = case shown="\"Check Input\", 默认" w100 {
      tunnel: w99 -> [_ _ _ w157 w158 w169 w182 w187]
      tunnel: [string[] ["Exit"] ("event queue out") string[] ["Check Input"] ("event queue out") w119 w157 w158 w169 w182 w187] -> w98
      tunnel: w96 -> [_ w107 _ w151 _ _ w181 w190]
      tunnel: w92 -> [w103 w112 w121 w156 w159 w161 w180 w188]
      tunnel: [w103 w112 w121 w156 w159 w160 w180 w188] -> w95
      tunnel: w94 -> [_ w109 _ _ _ _ _ _]
      tunnel: w93 -> [_ _ _ _ _ _ w178 _]
      frame "Exit" {
      }
      frame "Init" {
        w105 = FALSE ("Value")
        n9 = for {
          tunnel: w107 -> [w118] mode=indexing
          tunnel: [w117] -> w106 if=w117
          stop <- w117 stop-if-true
          n10 = Unbundle By Name(w118) -> ("NVH Configuration.NVH Station?"=w117:bool)
        }
        n11 = property on="Loop Stopped?" class="Bool (严格)"("Value"=w105) -> ()  [unwired: 2 in, 2 out]
        n12 = property on="Loop Stopped?" class="Bool (严格)"("Value"=w105) -> ()  [unwired: 2 in, 2 out]
        n13 = property on="Loop Stopped?" class="Bool (严格)"("Value"=w105) -> ()  [unwired: 2 in, 2 out]
        n14 = property on="Loop Stopped?" class="Bool (严格)"("Value"=w105) -> ()  [unwired: 2 in, 2 out]
        n15 = property on="Loop Stopped" class="Bool (严格)"("Value"=w105) -> ()  [unwired: 2 in, 2 out]
        n16 = Concatenate Strings(w109, " - All Stations Status" ("string")) -> (→"Main Title":string)
        n17 = case shown="真" w106 {
          frame False {
          }
          frame True {
            n18 = call <vilib>:"System Exec.vi"("run minimized? (F)"=TRUE, "wait until completion? (T)"=FALSE, "command line"="cmd /c \"C:\\Inalfa NVH System\\App\\Inalfa NVH System App.exe\"") -> ()  [unwired: 5 in, 4 out]
          }
        }
        "ms" <- 0.0 ("ms")
      }
      frame "Check Input", Default {
        n19 = event shown="[0] 超时" {
          selector: _ -> [_ _ _ _ _ _ _ _ _ _ _ _ _]
          dyn-events: _ -> [_ _ _ _ _ _ _ _ _ _ _ _ _]
          timeout: 100 -> [_ _ _ _ _ _ _ _ _ _ _ _ _]
          tunnel: [w128 string[] ["Part Configuration", "Check Input"] ("event queue out") string[] ["O'Scope Data", "Check Input"] ("event queue out") string[] ["NVH Status", "Check Input"] ("event queue out") string[] ["Update AP Data", "Check Input"] ("event queue out") _ _ _ _ _ _ string[] ["Sunshade Graphs", "Check Input"] ("event queue out") _] -> w119
          event Timeout {
            n20 = event-data() -> ()  [unwired: 1 in, 1 out]
            n21 = property on="Loop Stopped?" class="Bool (严格)"() -> ("Value"=w127:bool)  [unwired: 2 in, 2 out]
            n22 = property on="Loop Stopped?" class="Bool (严格)"() -> ("Value"=w125:bool)  [unwired: 2 in, 2 out]
            n23 = property on="Loop Stopped?" class="Bool (严格)"() -> ("Value"=w124:bool)  [unwired: 2 in, 2 out]
            n24 = property on="Loop Stopped?" class="Bool (严格)"() -> ("Value"=w123:bool)  [unwired: 2 in, 2 out]
            n25 = property on="Loop Stopped" class="Bool (严格)"() -> ("Value"=w122:bool)  [unwired: 2 in, 2 out]
            n26 = Compound Arithmetic op=AND(w127, w125, w124, w123, w122) -> (w126:bool)
            "All Stations Stopped" <- w126
            n27 = case shown="假" w126 {
              tunnel: [_ string[] ["Exit"] ("event queue out")] -> w128
              frame False {
              }
              frame True {
              }
            }
            n28 = Get Date/Time String() -> (date string=→"Date":string, time string=→"Time":string)  [unwired: 3 in]
          }
          event "Configuration": Value Change {
            n29 = event-data() -> ()  [unwired: 1 in, 5 out]
          }
          event "O'Scope Data": Value Change {
            n30 = event-data() -> ()  [unwired: 1 in, 5 out]
          }
          event "NVH Status": Value Change {
            n31 = event-data() -> ()  [unwired: 1 in, 6 out]
          }
          event "Update AP Data": Value Change {
            n32 = event-data() -> ()  [unwired: 1 in, 5 out]
          }
          event "All Stations": Value Change {
            n33 = event-data() -> ()  [unwired: 1 in, 3 out]
            n34 = property on="Main Tab Control" class="TabCtl (严格)"("Value"=T42."All Stations Status" ("Main Tab Control")) -> ()  [unwired: 2 in, 2 out]
          }
          event "st0": Value Change {
            n35 = event-data() -> ()  [unwired: 1 in, 3 out]
            n36 = property on="Main Tab Control" class="TabCtl (严格)"("Value"=T42."Station 0" ("Main Tab Control")) -> ()  [unwired: 2 in, 2 out]
          }
          event "st1": Value Change {
            n37 = event-data() -> ()  [unwired: 1 in, 3 out]
            n38 = property on="Main Tab Control" class="TabCtl (严格)"("Value"=T42."Station 1" ("Main Tab Control")) -> ()  [unwired: 2 in, 2 out]
          }
          event "st2": Value Change {
            n39 = event-data() -> ()  [unwired: 1 in, 3 out]
            n40 = property on="Main Tab Control" class="TabCtl (严格)"("Value"=T42."Station 2" ("Main Tab Control")) -> ()  [unwired: 2 in, 2 out]
          }
          event "st3": Value Change {
            n41 = event-data() -> ()  [unwired: 1 in, 3 out]
            n42 = property on="Main Tab Control" class="TabCtl (严格)"("Value"=T42."Station 3" ("Main Tab Control")) -> ()  [unwired: 2 in, 2 out]
          }
          event "Barcode": Value Change {
            n43 = event-data() -> ()  [unwired: 1 in, 3 out]
            n44 = property on="Main Tab Control" class="TabCtl (严格)"("Value"=T42."Barcode Station" ("Main Tab Control")) -> ()  [unwired: 2 in, 2 out]
          }
          event "Sunshade Graphs": Value Change {
            n45 = event-data() -> ()  [unwired: 1 in, 6 out]
          }
          event "Pretty Graphs": Value Change {
            n46 = event-data() -> ()  [unwired: 1 in, 3 out]
            n47 = property on="Main Tab Control" class="TabCtl (严格)"("Value"=T42."Eng Data Graphs" ("Main Tab Control")) -> ()  [unwired: 2 in, 2 out]
          }
        }
      }
      frame "O'Scope Data" {
        n48 = Index Array(array=w151) -> (element #1=w152:T9, element #2=w153:T9, element #3=w154:T9, element #4=w155:T9, element #5=w148:T9)  [unwired: 5 in]
        n49 = Unbundle By Name(w152) -> ("misc station config.Station Name"=w150:string)
        n50 = Unbundle By Name(w153) -> ("misc station config.Station Name"=w147:string)
        n51 = Unbundle By Name(w154) -> ("misc station config.Station Name"=w146:string)
        n52 = Unbundle By Name(w155) -> ("misc station config.Station Name"=w145:string)
        n53 = Unbundle By Name(w148) -> ("misc station config.Station Name"=w144:string)
        n54 = Build Array(w150, w147, w146, w145, w144) -> (w149:string[])
        n55 = call "EOL O'Scope Data.vi"("station names"=w149) -> ()  [unwired: 11 in]
      }
      frame "NVH Status" {
        n56 = call "EOL NVH Status HMI.vi"() -> ()  [unwired: 12 in]
      }
      frame "Update AP Data" {
        n57 = call <vilib>:"Read Characters From File.vi"("file path (dialog if empty)"="AP Data") -> ("character string"=w168:string)  [unwired: 5 in, 3 out]
        n58 = Unflatten From String(type=i16[][][] [], binary string=w168, error in (no error)=w161) -> (value=w166:i16[][][], error out=w160:errorcluster)  [unwired: 2 in, 1 out]
        n59 = for {
          tunnel: w166 -> [w170] mode=indexing
          shift-right: [w172] -> w164
          shift-left: i16[][] [] -> [w171]
          n60 = Build Array (concatenate)(w171, w170) -> (w172:i16[][])
        }
        n61 = Transpose 2D Array(2D array=w164) -> (transposed array=→"AP Data Graph":i16[][])
      }
      frame "Part Configuration" {
        n62 = call "Log In 2.0.vi"("required access level"=1, "Program Root Path"=w178) -> ("User Name Out"=w179:string, "Cancelled"=w176:bool, "passed"=w177:bool, "Level"=w173:i32)  [unwired: 5 in, 1 out]
        n63 = Compound Arithmetic op=AND(w177, invert w176) -> (w175:bool)
        n64 = case shown="真" w175 {
          tunnel: w181 -> [_ w186]
          tunnel: w179 -> [_ w185]
          tunnel: w178 -> [_ w184]
          tunnel: w173 -> [_ w183]
          frame False {
          }
          frame True {
            n65 = call "Seq Station Part Config.vi"("User Name"=w185, "Level"=w183, "station default states"=w186, "Base Path"=w184) -> ()  [unwired: 8 in]
          }
        }
      }
      frame "Sunshade Graphs" {
        n66 = Index Array(array=w190) -> (element #1=w193:T9, element #2=w194:T9)  [unwired: 2 in]
        n67 = Unbundle By Name(w193) -> ("misc station config.Station Name"=w192:string)
        n68 = Unbundle By Name(w194) -> ("misc station config.Station Name"=w191:string)
        n69 = Build Array(w192, w191) -> (w189:string[])
        n70 = call "EOL Sunshade O'Scope Data.vi"("station names"=w189) -> ()  [unwired: 11 in]
      }
    }
  }
  n71 = control-ref of="Red-Rabbit Mode 1"() -> (w38:refnum<vi>)
  n72 = control-ref of="Waveform Graph st 1"() -> (w33:refnum<vi>)
  n73 = control-ref of="Waveform Graph st 2"() -> (w18:refnum<vi>)
  n74 = control-ref of="Start Test st 1"() -> (w37:refnum<vi>)
  n75 = control-ref of="Abort Test st 1"() -> (w36:refnum<vi>)
  n76 = control-ref of="Manual Control st 1"() -> (w35:refnum<vi>)
  n77 = control-ref of="Route to Repair st 1"() -> (w34:refnum<vi>)
  n78 = control-ref of="Manual Control Repair"() -> (w27:refnum<vi>)
  n79 = control-ref of="Start Test Re"() -> (w26:refnum<vi>)
  n80 = control-ref of="Waveform Graph st 3"() -> (w8:refnum<vi>)
  n81 = control-ref of="Motion Data st 1"() -> (w1:refnum<vi>)
  n82 = control-ref of="Start Test st 2"() -> (w22:refnum<vi>)
  n83 = control-ref of="Abort Test st 2"() -> (w21:refnum<vi>)
  n84 = control-ref of="Manual Control st 2"() -> (w20:refnum<vi>)
  n85 = control-ref of="Route to Repair st 2"() -> (w19:refnum<vi>)
  n86 = control-ref of="Red-Rabbit Mode 2"() -> (w15:refnum<vi>)
  n87 = control-ref of="all station status st 1"() -> (w30:refnum<vi>)
  n88 = control-ref of="Individual Station Status st 1"() -> (w32:refnum<vi>)
  n89 = control-ref of="Motion Data st 2"() -> (w2:refnum<vi>)
  n90 = control-ref of="Sunshade Servo Data Close"() -> (w55:refnum<vi>)
  n91 = control-ref of="Sunshade Servo Data Open"() -> (w56:refnum<vi>)
  n92 = control-ref of="Waveform Graph st 0"() -> (w82:refnum<vi>)
  n93 = control-ref of="Red-Rabbit Mode 0"() -> (w69:refnum<vi>)
  n94 = control-ref of="Start Test st 3"() -> (w12:refnum<vi>)
  n95 = control-ref of="Abort Test st 3"() -> (w11:refnum<vi>)
  n96 = control-ref of="Manual Control st 3"() -> (w10:refnum<vi>)
  n97 = control-ref of="Route to Repair st 3"() -> (w9:refnum<vi>)
  n98 = control-ref of="Red-Rabbit Mode 3"() -> (w5:refnum<vi>)
  n99 = control-ref of="all station status st 2"() -> (w17:refnum<vi>)
  n100 = control-ref of="Individual Station Status st 2"() -> (w16:refnum<vi>)
  n101 = control-ref of="Exit Program"() -> (w52:refnum<vi>)
  n102 = control-ref of="Start Test st 0"() -> (w83:refnum<vi>)
  n103 = control-ref of="Abort Test st 0"() -> (w85:refnum<vi>)
  n104 = control-ref of="Manual Control st 0"() -> (w84:refnum<vi>)
  n105 = control-ref of="Route to Repair st 0"() -> (w86:refnum<vi>)
  n106 = control-ref of="all station status st 3"() -> (w7:refnum<vi>)
  n107 = control-ref of="Individual Station Status st 3"() -> (w6:refnum<vi>)
  n108 = control-ref of="Motion Data st 3"() -> (w3:refnum<vi>)
  n109 = control-ref of="Motion Data st 0"() -> (w80:refnum<vi>)
  n110 = control-ref of="all station status st 0"() -> (w79:refnum<vi>)
  n111 = control-ref of="Individual Station Status st 0"() -> (w81:refnum<vi>)
  n112 = Bundle By Name(cluster=w64, "ctl refs.Start Test"=w83, "ctl refs.Abort Test"=w85, "ctl refs.Manual Control"=w84, "ctl refs.Route to Repair"=w86, "ctl refs.Waveform Graph"=w82, "ctl refs.Motion Data"=w80, "ctl refs.all station status"=w79, "ctl refs.Individual Station Status"=w81, "ctl refs.exit program"=w52, "ctl refs.Sunshade Servo Data Open"=w56, "ctl refs.Sunshade Servo Data Close"=w55, "ctl refs.Red-Rabbit Mode"=w69) -> (w66:T9)
  n113 = Bundle By Name(cluster=w63, "ctl refs.Start Test"=w37, "ctl refs.Abort Test"=w36, "ctl refs.Manual Control"=w35, "ctl refs.Route to Repair"=w34, "ctl refs.Waveform Graph"=w33, "ctl refs.Motion Data"=w1, "ctl refs.all station status"=w30, "ctl refs.Individual Station Status"=w32, "ctl refs.exit program"=w52, "ctl refs.Sunshade Servo Data Open"=w56, "ctl refs.Sunshade Servo Data Close"=w55, "ctl refs.Red-Rabbit Mode"=w38) -> (w39:T9)
  n114 = Bundle By Name(cluster=w53, "ctl refs.Manual Control"=w27, "ctl refs.exit program"=w52, "ctl refs.Start Test"=w26) -> (w28:T9)
  n115 = Bundle By Name(cluster=w54, "ctl refs.Start Test"=w12, "ctl refs.Abort Test"=w11, "ctl refs.Manual Control"=w10, "ctl refs.Route to Repair"=w9, "ctl refs.Waveform Graph"=w8, "ctl refs.Motion Data"=w3, "ctl refs.all station status"=w7, "ctl refs.Individual Station Status"=w6, "ctl refs.exit program"=w52, "ctl refs.Sunshade Servo Data Open"=w56, "ctl refs.Sunshade Servo Data Close"=w55, "ctl refs.Red-Rabbit Mode"=w5) -> (w4:T9)
  n116 = Bundle By Name(cluster=w58, "ctl refs.Start Test"=w22, "ctl refs.Abort Test"=w21, "ctl refs.Manual Control"=w20, "ctl refs.Route to Repair"=w19, "ctl refs.Waveform Graph"=w18, "ctl refs.Motion Data"=w2, "ctl refs.all station status"=w17, "ctl refs.Individual Station Status"=w16, "ctl refs.exit program"=w52, "ctl refs.Sunshade Servo Data Open"=w56, "ctl refs.Sunshade Servo Data Close"=w55, "ctl refs.Red-Rabbit Mode"=w15) -> (w24:T9)
  n117 = control-ref of="All Stations Stopped"() -> (w61:refnum<vi>)
  n118 = control-ref of="ms"() -> (w67:refnum<vi>)
  n119 = call "EOL Analog Data Acquisition v1.1.vi"("ms"=w67, "error in"=w51, "Exit Refnum"=w61) -> ("error out"=w60:errorcluster)  [unwired: 8 in]
  n120 = control-ref of="Repair Station:"() -> (w29:refnum<vi>)
  n121 = Unbundle By Name(w39) -> ("misc station config.Station Name"=w40:string)
  n122 = Unbundle By Name(w66) -> ("misc station config.Station Name"=w68:string)
  n123 = Unbundle By Name(w4) -> ("misc station config.Station Name"=w13:string)
  n124 = Unbundle By Name(w24) -> ("misc station config.Station Name"=w23:string)
  n125 = call "test exe main.vi"("error in"=w51, "HWcurrent limt"=sgl 1.0, "Main State Cluster"=w24) -> ("error out"=w59:errorcluster)  [unwired: 8 in]
  n126 = call "test exe main.vi"("error in"=w51, "HWcurrent limt"=sgl 1.0, "Main State Cluster"=w39) -> ("error out"=w65:errorcluster)  [unwired: 8 in]
  n127 = call "repair main.vi"("error in"=w51, "repair station config"=w28, "repair status indicator"=w29) -> ("error out"=w49:errorcluster)  [unwired: 8 in]
  n128 = call "test exe main.vi"("CustormMode"=FALSE, "error in"=w51, "HWcurrent limt"=sgl 0.8, "Main State Cluster"=w66) -> ("error out"=w75:errorcluster)  [unwired: 7 in]
  n129 = call "test exe main.vi"("error in"=w51, "HWcurrent limt"=sgl 1.0, "Main State Cluster"=w4) -> ("error out"=w50:errorcluster)  [unwired: 8 in]
  n130 = property on="st1" class="Bool"("BoolText.Text"=w40) -> ()  [unwired: 2 in, 2 out]
  n131 = property on="st0" class="Bool"("BoolText.Text"=w68) -> ()  [unwired: 2 in, 2 out]
  n132 = property on="st3" class="Bool"("BoolText.Text"=w13) -> ()  [unwired: 2 in, 2 out]
  n133 = property on="st2" class="Bool"("BoolText.Text"=w23) -> ()  [unwired: 2 in, 2 out]
  n134 = Merge Errors(w60, w73, w75, w65, w59, w50, w49) -> (w74:errorcluster)
  n135 = control-ref of="st1"() -> (w47:refnum<vi>)
  n136 = control-ref of="st3"() -> (w45:refnum<vi>)
  n137 = control-ref of="st2"() -> (w46:refnum<vi>)
  n138 = control-ref of="NVH Status"() -> (w43:refnum<vi>)
  n139 = disable-structure shown="默认" {
    disable-tunnel: w74 -> [_ _]
    frame condition #0 (active) {
      n140 = local write "Exit Program"(FALSE ("Exit Program")) -> ()
    }
    frame condition #1 {
      n141 = Quit LabVIEW(quit? (T)=TRUE) -> ()
    }
  }
  n142 = Build Array(w47, w46, w45, w43) -> (w44:refnum<vi>[])
  n143 = for {
    tunnel: w44 -> [w198] mode=indexing
    tunnel: bool[] [FALSE, FALSE, FALSE, FALSE] -> [w197] mode=indexing
    n144 = property class="Bool"(reference=w198, "Visible"=w197) -> ()  [unwired: 1 in, 2 out]
  }
